vi "PPT Server.vi"(11 "DVR In":refnum<data-value>) -> (3 "DVR Out":refnum<data-value>)   [LabVIEW 2016]
uses:
  Data/Nicholas Data.lvclass
  <vilib>/MSR Consulting, LLC/Devices/PPT/PPT.lvclass
  C:/Program Files (x86)/National Instruments/LabVIEW 2016/vi.lib/MSR Consulting, LLC/Devices/Configurable Device/Configurable Device.lvclass
  Session/Raw FPGA/FPGA Session.lvclass
  C:/Program Files (x86)/National Instruments/LabVIEW 2016/vi.lib/MSR Consulting, LLC/General Reuse/Session APIs/_Session Fwk/Session - Root.lvclass
  <vilib>/MSR Consulting, LLC/General Reuse/Session APIs/Session Log/System Log.lvclass
  <vilib>/MSR Consulting, LLC/General Reuse/Session APIs/File Access/Config Data/Config Data.lvclass
  Session/Session/FPGA Serial.lvclass
  <vilib>/MSR Consulting, LLC/General Reuse/Session APIs/File Access/Config Data/Config Data.lvclass/Config Data.ctl
  <vilib>/MSR Consulting, LLC/General Reuse/Session APIs/Session Log/System Log.lvclass/System Log.ctl
  <vilib>/Platform/TimedLoop/XDataNode/timing_clust.ctl
  <vilib>/Platform/TimedLoop/XDataNode/nitl_modes.ctl
  <vilib>/Platform/TimedLoop/XDataNode/wakeup.ctl
  <vilib>/MSR Consulting, LLC/Devices/Configurable Device/Configurable Device.lvclass/Configurable Device.ctl
  <vilib>/MSR Consulting, LLC/General Reuse/Data/Array Data/Single 1-D/Single_Array.lvclass
  Data/Nicholas Data.lvclass/Nicholas Data.ctl
  <vilib>/MSR Consulting, LLC/Devices/Configurable Device/Write ID.vi
  Session/Session/Write FPGA Session.vi
  <vilib>/MSR Consulting, LLC/General Reuse/Session APIs/Serial/Public/Accessors/Write Sys Log.vi
  Data/Write PPT Data.vi
  <vilib>/MSR Consulting, LLC/General Reuse/Session APIs/File Access/Config Data/Accessors/Write Cfg Path.vi
  <vilib>/MSR Consulting, LLC/General Reuse/Session APIs/Session Log/Accessors/Write Main Path.vi
  <vilib>/Platform/TimedLoop/XDataNode/XDataNode.xnode
  <vilib>/MSR Consulting, LLC/General Reuse/Session APIs/_Session Fwk/Session - Root.lvclass
  <vilib>/Platform/TimedLoop/XDataNode/XDNodeRunTimeDep.lvlib
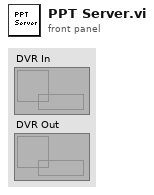
[diagram p1: front panel]
types:
  T1 = typedef "Session - Root.lvclass/Session Handle.ctl" = refnum<data-value>
  T2 = typedef "XDNodeRunTimeDep.lvlib/timing_clust.ctl" = cluster{"Expected End [f-1]":u64, "Actual End [f-1]":u64, "Finished Late? [f-1]":bool, "Expected End [i-1]":u64, "Actual End [i-1]":u64, "Finished Late? [i-1]":bool, "Expected Start [i]":u64, "Actual Start [i]":u64, "Expected Start [f]":u64, "Actual Start [f]":u64, "Source Name":string, "Structure Name":string, "Period":i64, "Deadline":i64, "Offset":i64, "Start":i64, "Priority":i32, "Timeout":i32, "Mode":T3, "Wakeup Reason":T4, "Error":errorcluster, "Source Type":string, "Secondary Source Type":string, "Global End Time":u64, "Global Start Time":u64, "Frame Duration":u64, "Iteration Duration":u64, "Assigned CPU":i32, "I/O Scan Engine Mode":u32}
  T3 = typedef "XDNodeRunTimeDep.lvlib/nitl_modes.ctl" = enum32{"No Change", "Process missed periods, maintain original phase", "Discard missed periods, maintain original phase", "Process missed periods, ignore original phase", "Discard missed periods, ignore original phase"}
  T4 = typedef "XDNodeRunTimeDep.lvlib/wakeup.ctl" = enum32{"Normal", "Aborted", "Asynchronous wakeup", "Timing source error", "Timed loop error", "Timeout"}
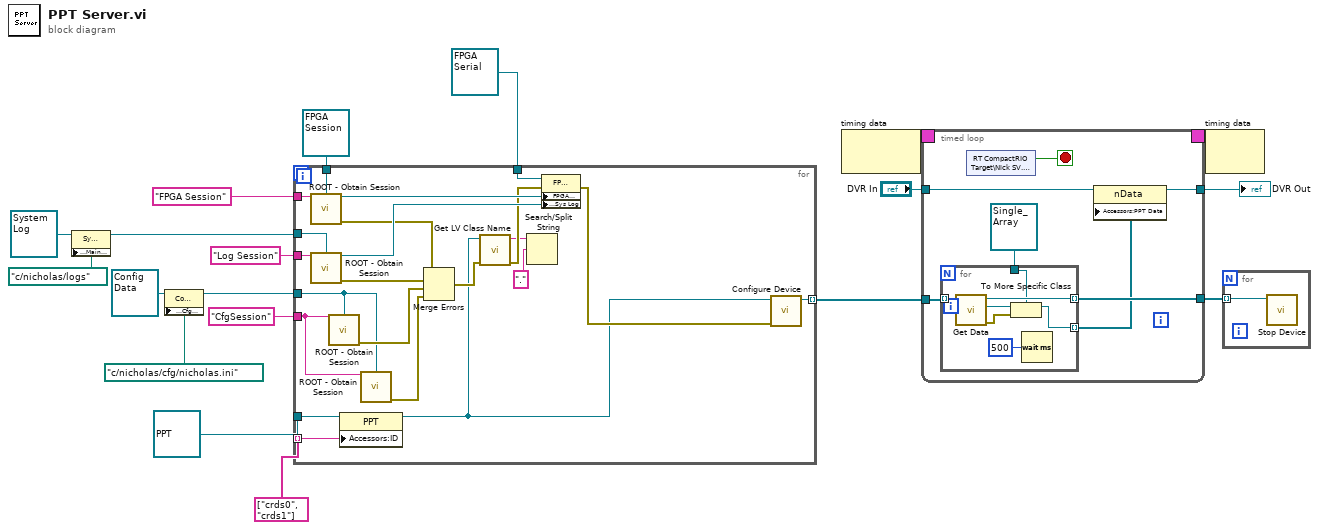
[diagram p0: block diagram]
diagram:
  n1 = property class="Sys Log"(reference=refnum<class "System Log.lvclass"> refnum ("Sys Log"), "Accessors:Main Path"=path "c:/nicholas/logs" ("Main Path")) -> (reference out=w10:refnum<class "System Log.lvclass">)  [unwired: 1 in, 1 out]
  n2 = property class="Config Data"(reference=refnum<class "Config Data.lvclass"> refnum ("Config Data"), "Accessors:Cfg Path"=path "c:/nicholas/cfg/nicholas.ini" ("Cfg Path")) -> (reference out=w11:refnum<class "Config Data.lvclass">)  [unwired: 1 in, 1 out]
  n3 = for {
    tunnel: w10 -> [w41]
    tunnel: "Log Session" ("Session Name ()") -> [w40]
    tunnel: refnum<class "FPGA Session.lvclass"> refnum ("FPGA Session") -> [w39]
    tunnel: "FPGA Session" ("Session Name ()") -> [w38]
    tunnel: w11 -> [w25]
    tunnel: "CfgSession" ("Session Name ()") -> [w26]
    tunnel: refnum<class "FPGA Serial.lvclass"> refnum ("FPGA Serial.lvclass") -> [w36]
    tunnel: string[] ["crds0", "crds1"] -> [w23] mode=indexing
    tunnel: refnum<class "PPT.lvclass"> refnum ("PPT") -> [w22]
    tunnel: [w20] -> w5 mode=indexing
    n4 = call <vilib>:"ROOT - Obtain Session.vi"("Session Name ()"=w38, "OBJ - Session"=w39) -> ("Session Handle"=w37:T1, "error out"=w34:errorcluster)  [unwired: 11 in, 1 out]
    n5 = call <vilib>:"ROOT - Obtain Session.vi"("Session Name ()"=w40, "OBJ - Session"=w41) -> ("Session Handle"=w35:T1, "error out"=w33:errorcluster)  [unwired: 11 in, 1 out]
    n6 = call <vilib>:"ROOT - Obtain Session.vi"("Session Name ()"=w26, "OBJ - Session"=w25) -> ("error out"=w32:errorcluster)  [unwired: 11 in, 2 out]
    n7 = property class="PPT"(reference=w22, "Accessors:ID"=w23) -> (reference out=w21:refnum<class "PPT.lvclass">)  [unwired: 1 in, 1 out]
    n8 = call <vilib>:"ROOT - Obtain Session.vi"("Session Name ()"=w26, "OBJ - Session"=w25) -> ("error out"=w24:errorcluster)  [unwired: 11 in, 2 out]
    n9 = Merge Errors(w34, w33, w32, w24) -> (w30:errorcluster)
    n10 = call <vilib>:"Get LV Class Name.vi"("error in (no error)"=w30, "object"=w21) -> ("error out"=w29:errorcluster, "class name"=w27:string)  [unwired: 8 in]
    n11 = Search/Split String(string=w27, search string/char (-)="." ("regular expression")) -> ()  [unwired: 1 in, 3 out]
    n12 = property class="FPGA Serial.lvclass"(reference=w36, error in=w29, "FPGA Session"=w37, "Public:Accessors:Sys Log"=w35) -> (error out=w31:errorcluster)  [unwired: 1 out]
    n13 = call-dynamic "Configure Device.vi"("error in"=w31, "PPT in"=w21) -> ("PPT out"=w20:refnum<class "PPT.lvclass">)  [unwired: 6 in, 3 out]
  }
  n14 = node-c288() -> (w7:T2)  [unwired: 1 in]
  n15 = timed-loop {
    tunnel: w5 -> [w48]
    tunnel: [w47] -> w2
    timing: w7 -> [_]
    timing-out: [_] -> w6
    tunnel: "DVR In" -> [w45]
    tunnel: [w43] -> w3
    stop <- w46 stop-if-true
    n16 = for {
      tunnel: w48 -> [w55] mode=indexing
      tunnel: [w54] -> w47 mode=indexing
      tunnel: refnum<class "Single_Array.lvclass"> refnum ("Base Data Lib:[SGL]") -> [w52]
      tunnel: [w51] -> w42 mode=indexing
      n17 = call-dynamic "Get Data.vi"("Cfg Dev in"=w55) -> ("error out"=w50:errorcluster, "Data"=w53:refnum<class "Data.lvclass">, "Cfg Dev out"=w54:refnum<class "PPT.lvclass">)  [unwired: 8 in]
      n18 = To More Specific Class(target class=w52, reference=w53, error in=w50) -> (specific class reference=w51:refnum<class "Single_Array.lvclass">)  [unwired: 1 out]
      n19 = Wait (ms)(milliseconds to wait=u32 500) -> ()  [unwired: 1 out]
    }
    n20 = shared-variable "RT CompactRIO Target\\Nick SV.lvlib\\Stop"() -> (w46:bool)  [unwired: 1 in, 1 out]
    n21 = property class="nData"(reference=w45, "Accessors:PPT Data"=w42) -> (reference out=w43:refnum<data-value>)  [unwired: 1 in, 1 out]
  }
  "DVR Out" <- w3
  n22 = node-c288(w6) -> ()  [unwired: 1 out]
  n23 = for {
    tunnel: w2 -> [w58] mode=indexing
    n24 = call-dynamic "Stop Device.vi"("Cfg Dev in"=w58) -> ()  [unwired: 9 in, 2 out]
  }
